vi "CreateRoomWalls.vi"(8 "error in (no error)":errorcluster, 10 "DirectionsList":T2[](array[typedef]), 11 "MazeGame in":refnum<class "MazeGame.lvclass">) -> (0 "error out":errorcluster, 2 "RoomWallsList":T1[](array[typedef]), 3 "MazeGame out":refnum<class "MazeGame.lvclass">)   [LabVIEW 2020, in "FactoryMethod.lvlib" / "NoParametrizedFactoryMethod.lvlib" / "MazeGame.lvclass"]
uses:
  MazeGame.lvclass
  GoFcommonClasses/Direction.ctl
  TypeDef/RoomElement.ctl
  GoFcommonClasses/MazeSite/MazeSite.lvclass
  GoFcommonClasses/ConcreteMazeSite/Wall/Wall.lvclass
  E:/GitHub/Design-Patterns-GoF_-_NI-LV/Creational/GoFcommonClasses/MazeSite/MazeSite.lvclass
  GoFcommonClasses/ConcreteMazeSite/Room/Room.lvclass
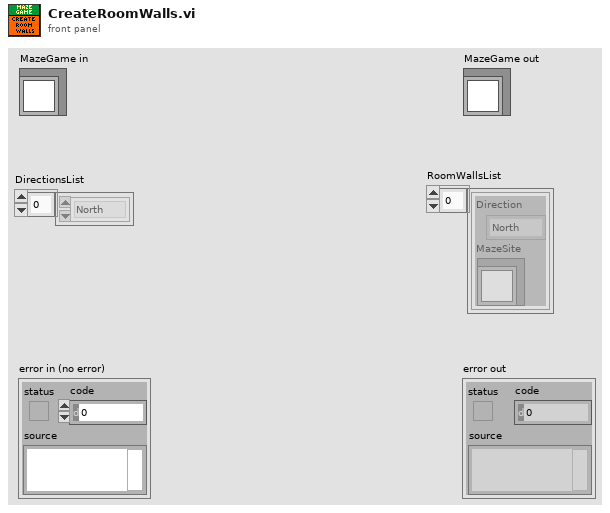
[diagram p1: front panel]
types:
  T1 = typedef "Room.lvclass/RoomElement.ctl" = cluster{"Direction":T2, "MazeSite":refnum<class "MazeSite.lvclass">}
  T2 = typedef "Direction.ctl" = enum32{"North", "South", "East", "West"}
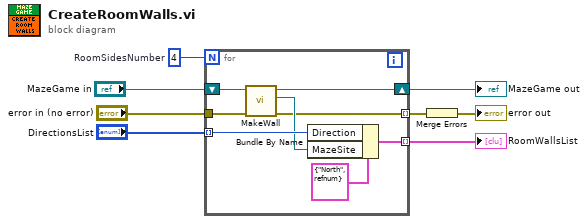
[diagram p0: block diagram]
diagram:
  w3 = 4  # RoomSidesNumber
  n1 = for {
    N: w3 -> [_]
    tunnel: "DirectionsList" -> [w16] mode=indexing
    tunnel: [w15] -> w5 mode=indexing
    tunnel: "error in (no error)" -> [w13]
    tunnel: [w12] -> w6 mode=indexing
    shift-right: [w9] -> w1
    shift-left: "MazeGame in" -> [w10]
    n2 = call-dynamic "MakeWall.vi"("error in (no error)"=w13, "MazeGame in"=w10) -> ("error out"=w12:errorcluster, "Wall"=w14:refnum<class "Wall.lvclass">, "MazeGame out"=w9:refnum<class "MazeGame.lvclass">)  [unwired: 7 in]
    n3 = Bundle By Name(cluster=T1 {"Direction"=enum."North", "MazeSite"=refnum} ("RoomElement"), "Direction"=w16, "MazeSite"=w14) -> (w15:T1)
  }
  "MazeGame out" <- w1
  "RoomWallsList" <- w5
  n4 = Merge Errors(w6) -> (→"error out":errorcluster)
